vi "GenerateStatisticData.vi"(11 "Num of Rows":i32=25) -> (3 "Output Array":string[][](array[string]))   [LabVIEW 2023]
uses:
  <vilib>/Utility/file.llb/Write Delimited Spreadsheet (string).vi
panel:
  in  "Sorted":bool
  # "Генерира Num of Rows x 3 на брой редове в 6 колони с произволни числа\nЧислата са \"уникални\" само в масив с размерност 3 х 6."
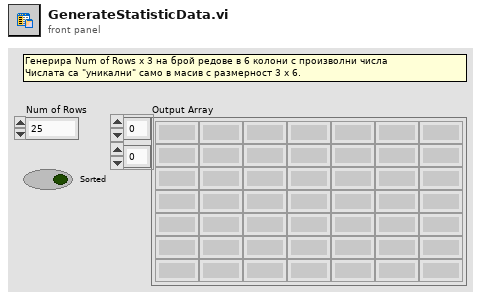
[diagram p1: front panel]
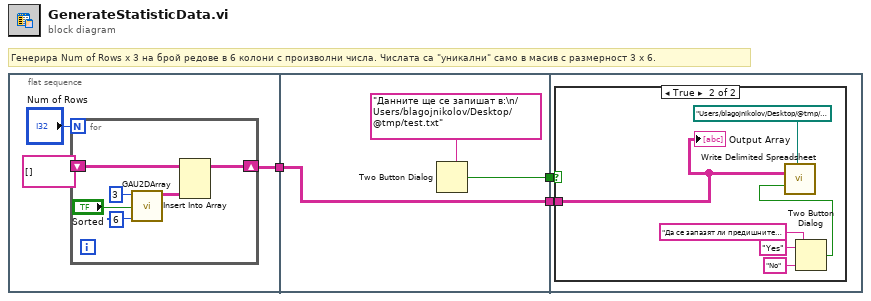
[diagram p0: block diagram]
diagram:
  # "Генерира Num of Rows x 3 на брой редове в 6 колони с произволни числа. Числата са \"уникални\" само в масив с размерност 3 х 6."
  n1 = flat-sequence {
    tunnel: [w5] -> w3
    tunnel: w3 -> [w13]
    tunnel: [w14] -> w2
    tunnel: [w13] -> w1
    tunnel: w2 -> [w17]
    tunnel: w1 -> [w16]
    frame #0 {
      n2 = for {
        N: "Num of Rows" -> [_]
        shift-right: [w9] -> w5
        shift-left: string[][] [] -> [w8]
        n3 = call "GAU2DArray.vi"("Colums"=6, "Sorted"="Sorted", "Rows"=3) -> ("2D String Array"=w10:string[][])  [unwired: 6 in, 2 out]
        n4 = Insert Into Array(array=w8, new element=w10) -> (w9:string[][])  [unwired: 2 in]
      }
    }
    frame #1 {
      n5 = Two Button Dialog(message="Данните ще се запишат в:\n/Users/blagojnikolov/Desktop/@tmp/test.txt") -> (T button?=w14:bool)  [unwired: 2 in]
    }
    frame #2 {
      n6 = case shown="True" w17 {
        tunnel: w16 -> [_ w22]
        frame False {
        }
        frame True {
          n7 = Two Button Dialog(message="Да се запазят ли предишните данни ?\n", 1:"No" ("F button name (\"Cancel\")"), 2:"Yes" ("T button name (\"OK\")")) -> (T button?=w18:bool)
          n8 = call-poly <vilib>:"Write Delimited Spreadsheet.vi"("file path (dialog if empty)"=path "/Users/blagojnikolov/Desktop/@tmp/test.txt", "2D data"=w22, "append to file? (new file:F)"=w18) -> ()  [unwired: 11 in, 2 out]
          "Output Array" <- w22
        }
      }
    }
  }
